vi "Seek_Operation_SUB_VI.vi"(0 "connection ID":refnum<k5>, 1 "Response ID":u8=68, 9 "Operation Message ID":i32=67, 11 "Error in":errorcluster, 12 "Operation Message Length":i32) -> (4 "connection ID out":refnum<k5>, 10 "End frequency and Time Stamp":string, 15 "error out":errorcluster)   [LabVIEW 2017]
panel:
  # "OUTPUT"
  # "INPUT"
  # "REQ"
  # "RES"
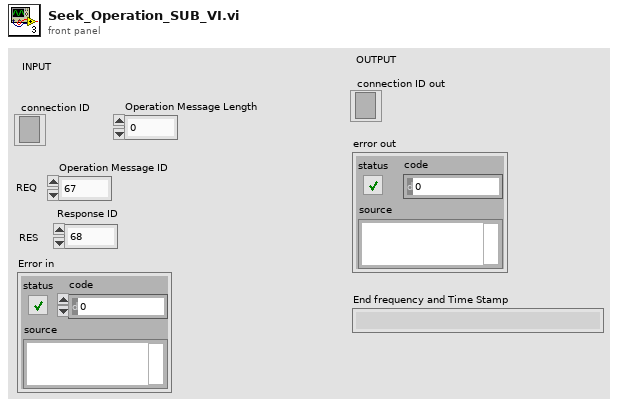
[diagram p1: front panel]
types:
  T1 = cluster{"Seek Request Message Length to DB ":i32, "Seek Request Message ID to DB":i32}
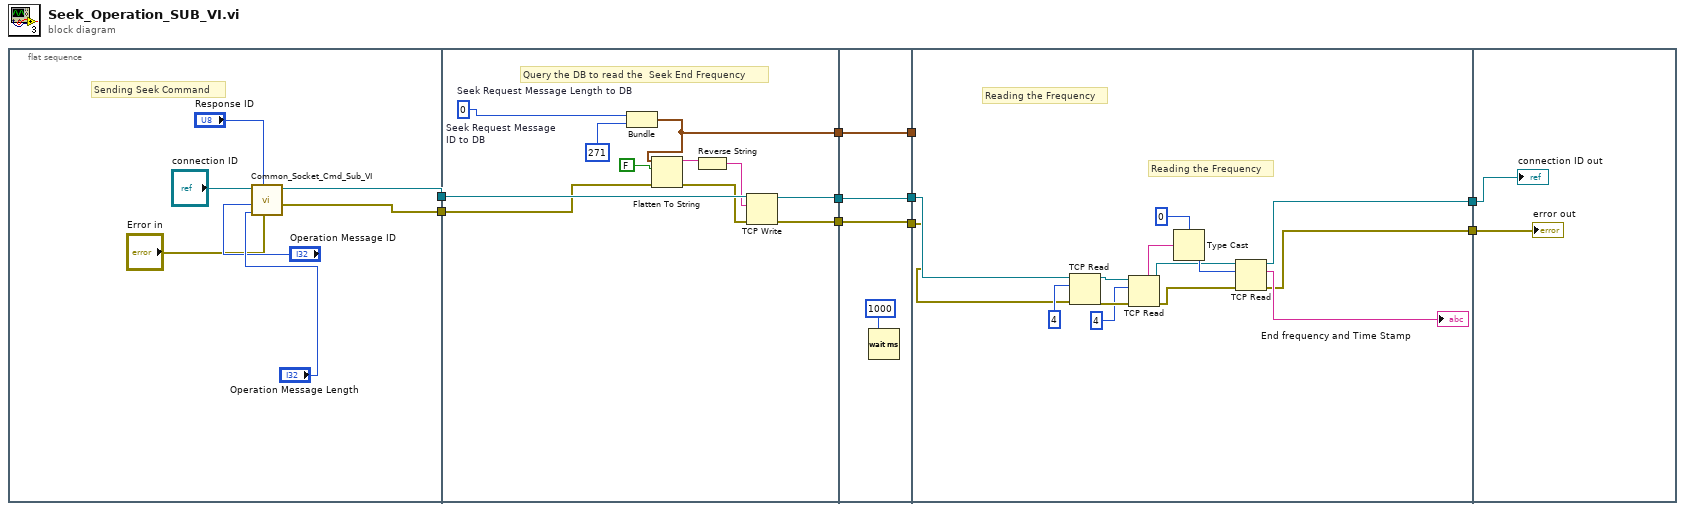
[diagram p0: block diagram]
diagram:
  n1 = flat-sequence {
    tunnel: [w17] -> w10
    tunnel: [w16] -> w3
    tunnel: w10 -> [w28]
    tunnel: [w21] -> w9
    tunnel: [w20] -> w8
    tunnel: [w19] -> w7
    tunnel: w3 -> [w24]
    tunnel: w9 -> [w30]
    tunnel: w8 -> [w31]
    tunnel: [w31] -> w6
    tunnel: [w30] -> w5
    tunnel: [w29] -> w4
    tunnel: w7 -> [w29]
    tunnel: [w36] -> w2
    tunnel: [w35] -> w1
    tunnel: w6 -> [w34]
    tunnel: w5 -> [w33]
    tunnel: w4 -> [_]
    tunnel: w2 -> [w48]
    tunnel: w1 -> [w47]
    frame #0 {
      # "Sending Seek Command"
      n2 = call "Common_Socket_Cmd_Sub_VI.vi"("Common Socket Error in"="Error in", "Response ID 1"="Response ID", "Operation Message Length 1"="Operation Message Length", "Operation Message ID 1"="Operation Message ID", "connection ID"="connection ID") -> ("error out"=w16:errorcluster, "connection ID"=w17:refnum<k5>)  [unwired: 4 in, 1 out]
    }
    frame #1 {
      w26 = 271  # Seek Request Message ID to DB
      w27 = 0  # Seek Request Message Length to DB
      # "Query the DB to read the  Seek End Frequency"
      n3 = Bundle("Seek Request Message Length to DB"=w27, "Seek Request Message ID to DB"=w26) -> (w19:T1)  [unwired: 1 in]
      n4 = Flatten To String(anything=w19, prepend array or string size? (T)=FALSE, error in (no error)=w24) -> (data string=w25:string, error out=w22:errorcluster)  [unwired: 1 in, 1 out]
      n5 = Reverse String(1:w25) -> (0:w23:string)
      n6 = TCP Write(connection ID=w28, data in=w23, error in (no error)=w22) -> (connection ID out=w20:refnum<k5>, error out=w21:errorcluster)  [unwired: 1 in, 1 out]
    }
    frame #2 {
      n7 = Wait (ms)(milliseconds to wait=u32 1000) -> ()  [unwired: 1 out]
    }
    frame #3 {
      # "Reading the Frequency"
      # "Reading the Frequency"
      n8 = TCP Read(connection ID=w34, bytes to read=4, error in (no error)=w33) -> (connection ID out=w45:refnum<k5>, error out=w44:errorcluster)  [unwired: 2 in, 1 out]
      n9 = TCP Read(connection ID=w45, bytes to read=4, error in (no error)=w44) -> (connection ID out=w39:refnum<k5>, data out=w42:string, error out=w38:errorcluster)  [unwired: 2 in]
      n10 = Type Cast(type=u8 0 ("bytes to read"), x=w42) -> (*(type *) &x=w40:u8)
      n11 = TCP Read(connection ID=w39, bytes to read=w40, error in (no error)=w38) -> (connection ID out=w36:refnum<k5>, data out=→"End frequency and Time Stamp":string, error out=w35:errorcluster)  [unwired: 2 in]
    }
    frame #4 {
      "error out" <- w47
      "connection ID out" <- w48
    }
  }
